vi "LED Output.vi"(8 "Pedestrian Light Display":T2, 9 "Traffic Light Display":T1, 11 "error in":errorcluster) -> (3 "error out":errorcluster)   [LabVIEW 2012]
doc: "DAQ assistant set up for use with the Traffic Lights LEDs"
uses:
  Controls/Pedestrian Light Display.ctl
  Controls/Traffic Light Display.ctl
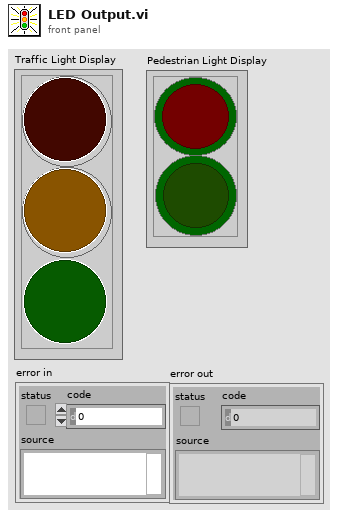
[diagram p1: front panel]
types:
  T1 = typedef "Traffic Light Display.ctl" = cluster{"RED":bool, "AMBER":bool, "GREEN":bool}
  T2 = typedef "Pedestrian Light Display.ctl" = cluster{"Red":bool, "Green":bool}
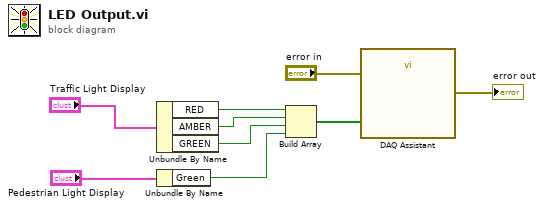
[diagram p0: block diagram]
diagram:
  n1 = Unbundle By Name("Traffic Light Display") -> ("RED"=w9:bool, "AMBER"=w8:bool, "GREEN"=w7:bool)
  n2 = Unbundle By Name("Pedestrian Light Display") -> ("Green"=w6:bool)
  n3 = Build Array(w9, w8, w7, w6) -> (w5:bool[])
  n4 = call "DAQ Assistant"("data"=w5, "error in"="error in") -> ("error out"=→"error out":errorcluster)  [unwired: 16 in, 1 out]
